vi "Save Logs.vi"(8 "Error In":errorcluster, 11 "EventLog in":refnum<class "LogsAbstract.lvclass">) -> (0 "Error Out":errorcluster, 3 "EventLog out":refnum<class "LogsAbstract.lvclass">)   [LabVIEW 2019, in "LogsAbstract.lvlib" / "LogsAbstract.lvclass"]
uses:
  LogsAbstract.lvclass
  LogsAbstract.lvclass/LogsAbstract.ctl
  8ebcb51d-6aa0-4ebd-80a8-675e538a3599.vi
  8ebcb51d-6aa0-4ebd-80a8-675e538a3599.vi/b87348bf-a6f8-4a0e-84d9-ac7e394ca3be.vi
  Accessors/Write LogPath.vi
  Accessors/Read LogPath.vi
  <vilib>/Utility/file.llb/Write Delimited Spreadsheet.vi
  <vilib>/Utility/file.llb/Write Delimited Spreadsheet (string).vi
  ea979658-2d34-4955-86e6-3a3c92514f7e.vi
  Classes/EventsAbstract/EventsAbstract.lvclass
  Classes/Event/Event.lvclass
  4b94c8d1-4b01-438e-b510-41d1fa3d74a3.vi
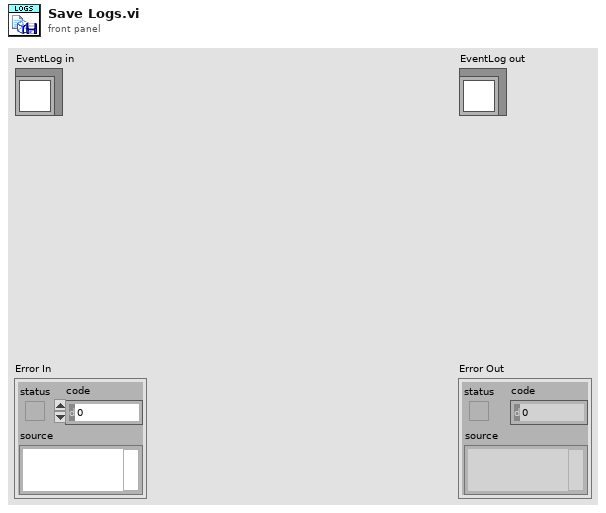
[diagram p1: front panel]
types:
  T1 = typedef "Event.lvclass/Event Classification.ctl" = enum16{"System Log", "test1", "test2", "test3"}
  T2 = typedef "LogsAbstract.lvlib/LogsAbstract.lvclass/Event Source.ctl" = enum16{"Unknown", "< --- Modules --- >", "Core", "< --- SubModules --- >", "Core -> EventLog", "Core -> ErrorLog"}
  T3 = cluster{"Date":string, "Time":string, "Description":string, "Comments":string, "Source":T2}
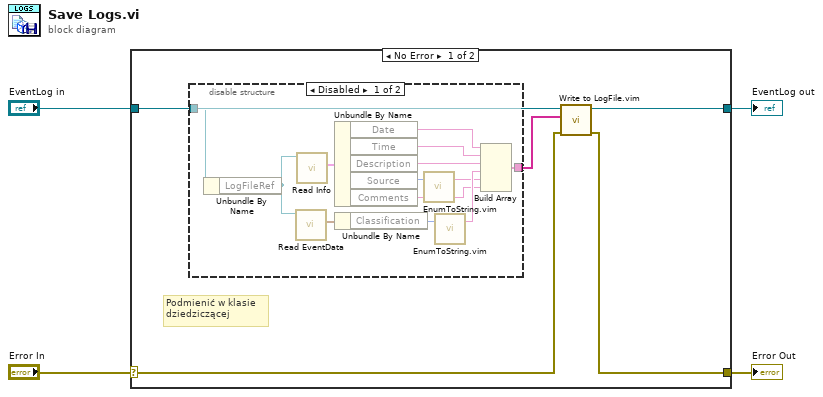
[diagram p0: block diagram]
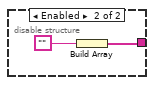
[diagram p2: hidden frame]
diagram:
  n1 = case shown="No Error" "Error In" {
    selector: "Error In" -> [w7 w26]
    tunnel: [w6 w26] -> w3
    tunnel: [w8 w25] -> w1
    tunnel: "EventLog in" -> [w9 w25]
    frame No Error {
      # "Podmienić w klasie\ndziedziczącej"
      n2 = disable-structure shown="Disabled" {
        disable-tunnel: w9 -> [w22 _]
        disable-tunnel: [w11 w23] -> w5
        frame Disabled {
          n3 = Unbundle By Name(w22) -> ("LogFileRef"=w21:refnum<file>)
          n4 = call "Read EventData.vi"("Event in"=w21) -> ("EventData"=w19:cluster{"Classification":T1})  [unwired: 8 in, 2 out]
          n5 = call "Read Info.vi"("EventsAbstract in"=w21) -> ("Info"=w20:T3)  [unwired: 8 in, 2 out]
          n6 = Unbundle By Name(w20) -> ("Date"=w17:string, "Time"=w16:string, "Description"=w15:string, "Source"=w13:T2, "Comments"=w12:string)
          n7 = Unbundle By Name(w19) -> ("Classification"=w18:T1)
          n8 = call "EnumToString.vim"("Enum"=w13) -> ("Enum Value"=w10:string)  [unwired: 16 in, 2 out]
          n9 = call "EnumToString.vim"("Enum"=w18) -> ("Enum Value"=w14:string)  [unwired: 16 in, 2 out]
          n10 = Build Array(w17, w16, w15, w14, w10, w12) -> (w11:string[])
        }
        frame Enabled {
          n11 = Build Array("") -> (w23:string[])
        }
      }
      n12 = call "Write to LogFile.vim"("Error In"=w7, "Data"=w5, "LogClass In"=w9) -> ("Error out"=w6:errorcluster, "LogClass Out"=w8:refnum<class "LogsAbstract.lvclass">)  [unwired: 7 in]
    }
    frame Error {
    }
  }
  "Error Out" <- w3
  "EventLog out" <- w1
